vi "Proxy_CheckP.vi"(8 "Data - O2":dbl format="%#_13g", 9 "Time":timestamp, 11 "Data - P":i16[](array[numeric])) -> (0 "O2 Valid?":bool, 1 "Data - O2":dbl format="%#_13g", 2 "Data - P":dbl[](array[numeric]), 3 "Times":timestamp[](array[timestamp]))   [LabVIEW 2019, in "Channel.lvlib" / "Serial.lvlib"]
uses:
  Serial.lvlib
  <vilib>/Analysis/NI_AALBase.lvlib
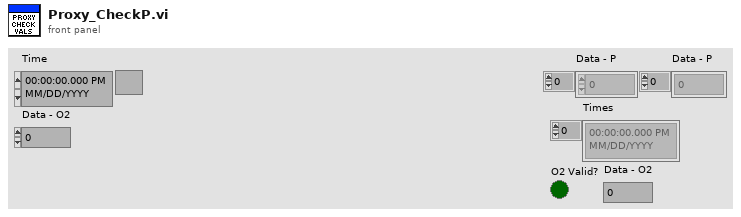
[diagram p1: front panel]
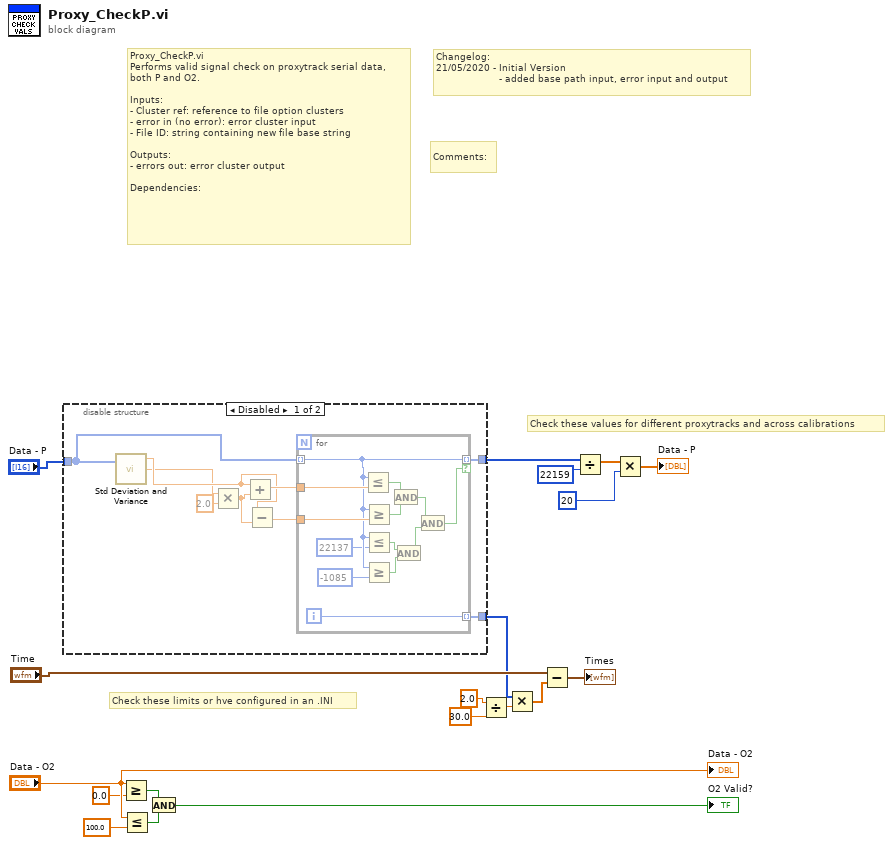
[diagram p0: block diagram]
diagram:
  # "Comments:"
  # "Changelog:\n21/05/2020 - Initial Version\n                     - added base path input, error input and output"
  # "Proxy_CheckP.vi\nPerforms valid signal check on proxytrack serial data,\nboth P and O2.\n\nInputs:\n- Cluster ref: reference to file option clusters\n- error in (no error): error cluster input\n- File ID: string containing new file base string\n\nOutputs:\n- errors out: error cluster output\n\nDependencies:"
  # "Check these limits or hve configured in an .INI"
  # "Check these values for different proxytracks and across calibrations"
  n1 = disable-structure shown="Disabled" {
    disable-tunnel: "Data - P" -> [w22 w42]
    disable-tunnel: [w21 w42] -> w15
    disable-tunnel: [w20 _] -> w10
    frame Disabled {
      n2 = call <vilib>:"Std Deviation and Variance.vi"("X"=w22) -> ("mean"=w24:dbl, "standard deviation"=w23:dbl)  [unwired: 1 in, 1 out]
      n3 = Multiply(x=w23, y=2.0) -> (x*y=w26:dbl)
      n4 = Add(x=w24, y=w26) -> (x+y=w27:dbl)
      n5 = Subtract(x=w24, y=w26) -> (x-y=w28:dbl)
      n6 = for {
        tunnel: w22 -> [w35] mode=indexing
        tunnel: w27 -> [w41]
        tunnel: w28 -> [w40]
        tunnel: [w35] -> w21 mode=indexing if=w36
        tunnel: [w29] -> w20 mode=indexing
        i -> [w29]
        n7 = Less Or Equal?(x=w35, y=w41) -> (x <= y?=w39:bool)
        n8 = Greater Or Equal?(x=w35, y=w40) -> (x >= y?=w38:bool)
        n9 = Less Or Equal?(x=w35, y=i16 22137) -> (x <= y?=w32:bool)
        n10 = Greater Or Equal?(x=w35, y=i16 -1085) -> (x >= y?=w31:bool)
        n11 = And(x=w39, y=w38) -> (x .and. y?=w37:bool)
        n12 = And(x=w32, y=w31) -> (x .and. y?=w30:bool)
        n13 = And(x=w37, y=w30) -> (x .and. y?=w36:bool)
      }
    }
    frame Enabled {
    }
  }
  n14 = Greater Or Equal?(x="Data - O2", y=0.0) -> (x >= y?=w6:bool)
  n15 = Less Or Equal?(x="Data - O2", y=100.0) -> (x <= y?=w7:bool)
  n16 = And(x=w6, y=w7) -> (x .and. y?=→"O2 Valid?":bool)
  n17 = Divide(x=2.0 ("y"), y=30.0) -> (x/y=w11:dbl)
  n18 = Multiply(x=w10, y=w11) -> (x*y=w9:dbl[])
  n19 = Subtract(x="Time", y=w9) -> (x-y=→"Times":timestamp[])
  n20 = Divide(x=w15, y=22159) -> (x/y=w17:dbl[])
  n21 = Multiply(x=w17, y=20) -> (x*y=→"Data - P":dbl[])
  "Data - O2" <- "Data - O2"
